vi "LvMPDC_SUB_convert_path2pathtext.vi"(10 "path":path) -> (2 "pathtext":string)   [LabVIEW 2012]
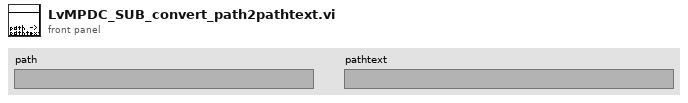
[diagram p1: front panel]
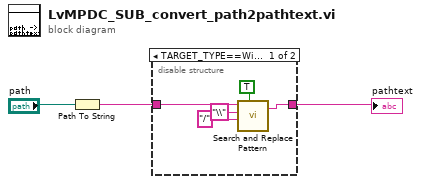
[diagram p0: block diagram]
diagram:
  n1 = Path To String(path="path") -> (string=w2:string)
  n2 = disable-structure shown="TARGET_TYPE==Windows" {
    disable-tunnel: w2 -> [w7 w9]
    disable-tunnel: [w4 w9] -> w1
    frame condition #0 (active) {
      n3 = call <vilib>:"Search and Replace Pattern.vi"("string"=w7, "regular expression (\"\")"="\\" ("regular expression (\"\")"), "replace string (\"\")"="/" ("replace string (\"\")"), "replace all? (F)"=TRUE) -> ("result string"=w4:string)  [unwired: 1 in, 1 out]
    }
    frame condition #1 {
    }
  }
  "pathtext" <- w1
